vi "Do Request.vi"(7 "Processing In":refnum<class "Processing.lvclass">, 11 "Test WebSocket Page Controller in":refnum<class "Test WebSocket Page Controller.lvclass">) -> (0 "error out":errorcluster, 5 "Processing":refnum<class "Processing.lvclass">)   [LabVIEW 2020, in "Test WebSocket Page Controller.lvclass"]
uses:
  Test WebSocket Page Controller.lvclass
  lv-http-util/HTTP Utils/Response/Response.lvclass
  lv-http-server/HTTP Server/Processing/Processing.lvclass
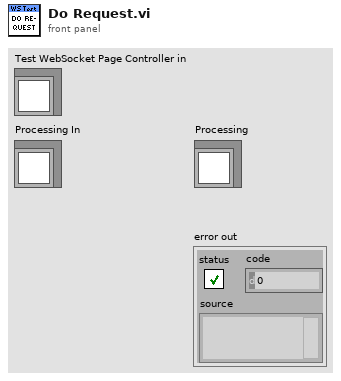
[diagram p1: front panel]
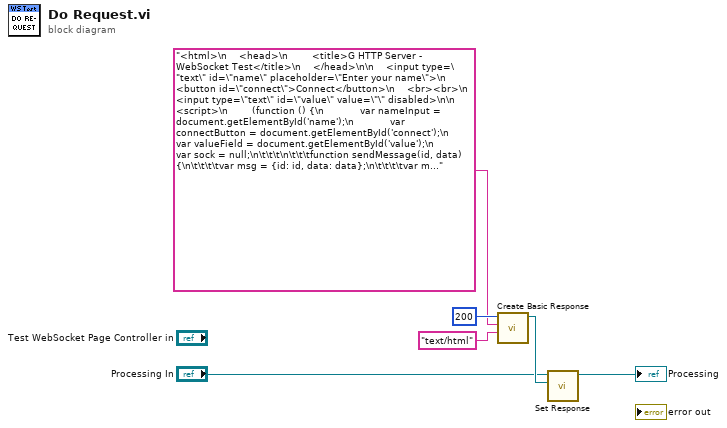
[diagram p0: block diagram]
diagram:
  n1 = call "Create Basic Response.vi"("Content-Type (text/plain)"="text/html", "Payload"="<html>\n    <head>\n        <title>G HTTP Server - WebSocket Test</title>\n    </head>\n\n    <input type=\"text\" id=\"name\" placeholder=\"Enter your name\">\n    <button id=\"connect\">Connect</button>\n    <br><br>\n    <input type=\"text\" id=\"value\" value=\"\" disabled>\n\n    <script>\n        (function () {\n            var nameInput = document.getElementById('name');\n            var connectButton = document.getElementById('connect');\n            var valueField = document.getElementById('value');\n            var sock = null;\n\t\t\t\n\t\t\tfunction sendMessage(id, data) {\n\t\t\t\tvar msg = {id: id, data: data};\n\t\t\t\tvar msgJSON = JSON.stringify(msg);\n\t\t\t\tsock.send(msgJSON);\n\t\t\t}\n\n            function onConnectClick(evt) {\n                connectButton.disabled = true;\n\n                sock = new WebSocket('ws://localhost:36987/ws');\n                sock.addEventListener('open', onConnect);\n                sock.addEventListener('close', onDisconnect);\n                sock.addEventListener('error', onError);\n                sock.addEventListener('message', onMessage);\n            }\n\n            function onConnect(evt) {\n                console.log('Connected!');\n\t\t\t\tsendMessage('sayhi', nameInput.value);\n            }\n\n            function onMessage(evt) {\n\t\t\t\tvar msg = JSON.parse(evt.data);\n\t\t\t\t\n                switch (msg.id) {\n                    case 'value':\n                        valueField.value = msg.data;\n                        break;\n                    \n                    default:\n                        console.log(evt);\n                        break;\n                }\n            }\n\n            function onDisconnect(evt) {\n                connectButton.disabled = false;\n            }\n\n            function onError(evt) {\n                console.log(evt);\n                connectButton.disabled = false;\n            }\n\n            connectButton.addEventListener('click', onConnectClick);\n        })();\n    </script>\n</html>", "Status Code"=u16 200) -> ("Response out"=w3:refnum<class "Response.lvclass">)  [unwired: 7 in, 1 out]
  n2 = call "Set Response.vi"("Response"=w3, "Processing in"="Processing In") -> ("Processing out"=→"Processing":refnum<class "Processing.lvclass">)  [unwired: 9 in]
